vi "Thread@ForeachStart__Parameter.vi"(1 "ParamterIn":string) -> (0 "ParamterOut":string)   [LabVIEW 2020]
uses:
  MainFrame/Global.vi
panel:
  in  "Thread Label":string(combo)
  in  "Confirm":bool
  # "Thread@ForeachStart $Label\nEX:\nVariable@VariableSet Var1,[aaa;bbb;ccc;ddd]\nThread@ForeachStart Loop\nThread@ForeachLoop Loop, Var1"
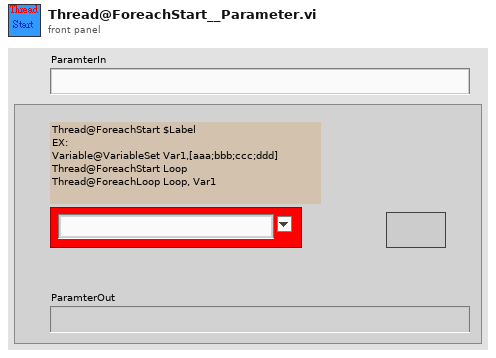
[diagram p1: front panel]
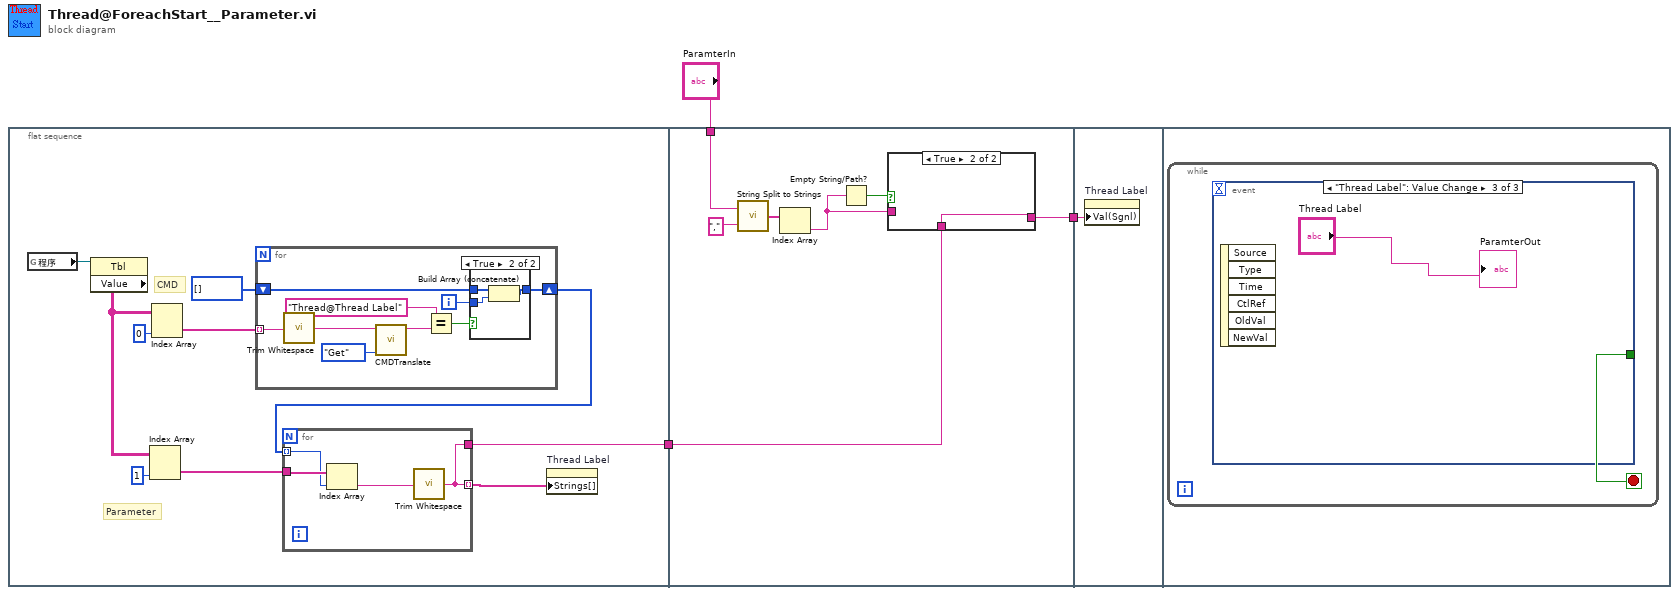
[diagram p0: block diagram]
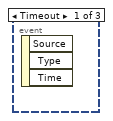
[diagram p4: hidden frame]
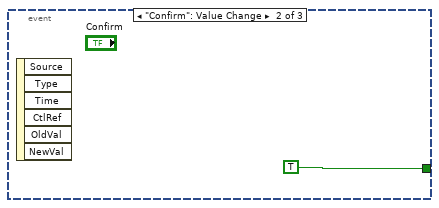
[diagram p5: hidden frame]
diagram:
  n1 = flat-sequence {
    tunnel: [w4] -> w1
    tunnel: "ParamterIn" -> [w35]
    tunnel: [w32] -> w2
    tunnel: w1 -> [w31]
    tunnel: w2 -> [w40]
    frame #0 {
      # "Parameter"
      # "CMD"
      n2 = global read "Global.vi" "程序"() -> (w13:refnum<vi>)
      n3 = property class="Tbl"(reference=w13) -> ("Value"=w10:string[][])  [unwired: 1 in, 2 out]
      n4 = Index Array(array=w10, index (col)=1 ("index (row)")) -> (element=w7:string[])  [unwired: 1 in]
      n5 = Index Array(array=w10, index (col)=0 ("index (row)")) -> (element=w9:string[])  [unwired: 1 in]
      n6 = for {
        tunnel: w9 -> [w19] mode=indexing
        shift-right: [w21] -> w6
        shift-left: i32[] [] -> [w23]
        i -> [w22]
        n7 = call <vilib>:"Trim Whitespace.vi"("string"=w19) -> ("trimmed string"=w18:string)  [unwired: 1 in]
        n8 = call "CMDTranslate.vi"("OP"=enum16{"Init", "Set", "Get", "GetInverse"}."Get", "CMDIn"=w18) -> ("CMDOut"=w20:string)  [unwired: 9 in]
        n9 = Equal?(x="Thread@Thread Label", y=w20) -> (x = y?=w24:bool)
        n10 = case shown="True" w24 {
          tunnel: w23 -> [w27 w30]
          tunnel: w22 -> [_ w29]
          tunnel: [w27 w28] -> w21
          frame False {
          }
          frame True {
            n11 = Build Array (concatenate)(w30, w29) -> (w28:i32[])
          }
        }
      }
      n12 = for {
        tunnel: w7 -> [w17]
        tunnel: w6 -> [w16] mode=indexing
        tunnel: [w15] -> w5 mode=indexing
        tunnel: [w15] -> w4
        n13 = Index Array(array=w17, index=w16) -> (element=w14:string)
        n14 = call <vilib>:"Trim Whitespace.vi"("string"=w14) -> ("trimmed string"=w15:string)  [unwired: 1 in]
      }
      n15 = property on="Thread Label" class="CmbBox"("Strings[]"=w5) -> ()  [unwired: 2 in, 2 out]
    }
    frame #1 {
      n16 = call "String Split to Strings.vi"("search string/char (-)"=",", "String"=w35) -> ("Array"=w37:string[])
      n17 = Index Array(array=w37) -> (element=w33:string)  [unwired: 1 in]
      n18 = Empty String/Path?(string/path=w33) -> (empty?=w34:bool)
      n19 = case shown="True" w34 {
        tunnel: w33 -> [w38 _]
        tunnel: [w38 w39] -> w32
        tunnel: w31 -> [_ w39]
        frame False {
        }
        frame True {
        }
      }
    }
    frame #2 {
      n20 = property on="Thread Label" class="CmbBox"("Val(Sgnl)"=w40) -> ()  [unwired: 2 in, 2 out]
    }
    frame #3 {
      n21 = while {
        stop <- w41 stop-if-true
        n22 = event shown="[2] \"Thread Label\": Value Change" {
          selector: _ -> [_ _ _]
          dyn-events: _ -> [_ _ _]
          timeout: _ -> [_ _ _]
          tunnel: [_ TRUE _] -> w41
          event Timeout {
            n23 = event-data() -> ()  [unwired: 1 in, 3 out]
          }
          event "Confirm": Value Change {
            n24 = event-data() -> ()  [unwired: 1 in, 6 out]
          }
          event "Thread Label": Value Change {
            n25 = event-data() -> ()  [unwired: 1 in, 6 out]
            "ParamterOut" <- "Thread Label"
          }
        }
      }
    }
  }
